vi "SVFA Magnitude and Phase to Real and Imaginary.vi"   [LabVIEW 2017]
doc: "Converts spectra from polar components to rectangular components. This conversion can reduce the computational power necessary to view and process spectra. Wire data to the <B>magnitude spectrum</B> and <B>phase spectrum</B> inputs to determine the polymorphic instance to use or manually select the instance."
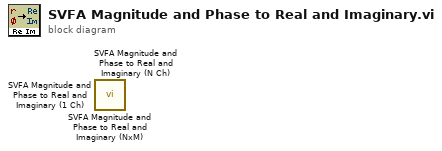
[diagram p0: block diagram]
diagram:
  n1 = call <vilib>:"SVFA Magnitude and Phase to Real and Imaginary (NxM).vi"() -> ()  [unwired: 14 in, 6 out]
  n2 = call <vilib>:"SVFA Magnitude and Phase to Real and Imaginary (N Ch).vi"() -> ()  [unwired: 14 in, 6 out]
  n3 = call <vilib>:"SVFA Magnitude and Phase to Real and Imaginary (1 Ch).vi"() -> ()  [unwired: 14 in, 6 out]
